vi "HFRR ADV v01.vi"() -> ()   [LabVIEW 2025] (continued)
        n280 = call "ELAPSED TIMER VI - Calibration.vi"("RESET"=w303, "PAUSE"=w303) -> ()  [unwired: 7 in, 3 out]
      }
      frame True {
        w306 = FALSE ("PAUSE")
        n281 = call "ELAPSED TIMER VI - Calibration.vi"("TARGET"=60.0, "RESET"=w306, "PAUSE"=w306) -> ("ELAPSED INDICATION"=w304:bool)  [unwired: 6 in, 2 out]
        n282 = case shown="False" w304 {
          frame False {
            n283 = local write "Friction Force Calibration Result Tab"(enum32{"Calibration Results", "Page 2"}."Calibration Results" ("Friction Force Calibration Result Tab")) -> ()
            n284 = property on="Friction Force Calibration Result Tab" class="TabCtl (strict)"("Visible"=FALSE) -> ()  [unwired: 2 in, 2 out]
          }
          frame True {
            n285 = stacked-sequence {
              frame #0 {
                n286 = local read "Friction"() -> (→"Friction cal":dbl)
                n287 = local write "run test Calibration"(FALSE ("run test Calibration")) -> ()
                n288 = local write "START TEMP"(FALSE ("START TEMP")) -> ()
              }
              frame #1 {
                n289 = Wait (ms)(milliseconds to wait=u32 1500) -> ()  [unwired: 1 out]
              }
              frame #2 {
                n290 = local write "Due Write"("VC;0") -> ()
              }
              frame #3 {
                n291 = Wait (ms)(milliseconds to wait=u32 1500) -> ()  [unwired: 1 out]
              }
              frame #4 {
                n292 = local write "Due Write"("VC;0") -> ()
              }
              frame #5 {
                n293 = property on="Friction Force Calibration Result Tab" class="TabCtl (strict)"("Visible"=TRUE) -> ()  [unwired: 2 in, 2 out]
                n294 = property on="Tab Control 6" class="TabCtl (strict)"("Visible"=FALSE) -> ()  [unwired: 2 in, 2 out]
              }
            }
          }
        }
      }
    }
    n295 = local read "Friction cal"() -> (w274:dbl)
    n296 = case shown="False" w278 {
      frame False {
        n297 = property on="Accept & Save" class="Bool (strict)"("DisabledEnum"=T20."Disabled" ("Disabled")) -> ()  [unwired: 2 in, 2 out]
        n298 = property on="Tab Control 5" class="TabCtl (strict)"("Value"=enum32{"OK", "NG"}."NG" ("Tab Control 5")) -> ()  [unwired: 2 in, 2 out]
      }
      frame True {
        n299 = property on="Accept & Save" class="Bool (strict)"("DisabledEnum"=T20."Enabled" ("Disabled")) -> ()  [unwired: 2 in, 2 out]
        n300 = property on="Tab Control 5" class="TabCtl (strict)"("Value"=enum32{"OK", "NG"}."OK" ("Tab Control 5")) -> ()  [unwired: 2 in, 2 out]
      }
    }
    n301 = Greater Or Equal?(x=w274, y="FF CAL EXCPTED VALUE") -> (x >= y?=w272:bool)
    n302 = case shown="False" w272 {
      selector: w272 -> [w285 w288]
      frame False {
        n303 = local write "FF PASS"(w285) -> ()
        n304 = local write "Friction Force result Tab"(enum32{"OK", "NG"}."NG" ("Friction Force result Tab")) -> ()
        n305 = property on="Accept & Save FF" class="Bool (strict)"("DisabledEnum"=T20."Disabled" ("Disabled")) -> ()  [unwired: 2 in, 2 out]
      }
      frame True {
        n306 = local write "Friction Force result Tab"(enum32{"OK", "NG"}."OK" ("Friction Force result Tab")) -> ()
        n307 = property on="Accept & Save FF" class="Bool (strict)"("DisabledEnum"=T20."Enabled" ("Disabled")) -> ()  [unwired: 2 in, 2 out]
        "FF PASS" <- w288
      }
    }
    n308 = local read "Quit"() -> (w284:bool)
  }
  n309 = while {
    stop <- w406 stop-if-true
    n310 = event shown="[13] \"Cal Password\": Value Change" {
      selector: _ -> [_ _ _ _ _ _ _ _ _ _ _ _ _ _ _ _ _ _ _ _ _ _ _ _ _ _ _ _ _ _ _ _ _ _ _ _ _ _ _ _ _ _ _ _ _ _ _ _ _ _ _ _ _ _ _ _ _]
      dyn-events: _ -> [_ _ _ _ _ _ _ _ _ _ _ _ _ _ _ _ _ _ _ _ _ _ _ _ _ _ _ _ _ _ _ _ _ _ _ _ _ _ _ _ _ _ _ _ _ _ _ _ _ _ _ _ _ _ _ _ _]
      timeout: 100 -> [_ _ _ _ _ _ _ _ _ _ _ _ _ _ _ _ _ _ _ _ _ _ _ _ _ _ _ _ _ _ _ _ _ _ _ _ _ _ _ _ _ _ _ _ _ _ _ _ _ _ _ _ _ _ _ _ _]
      tunnel: [FALSE FALSE FALSE _ FALSE _ _ _ _ _ _ _ _ _ _ _ _ _ _ _ _ _ _ _ _ _ _ _ _ _ _ _ _ _ _ _ _ _ _ _ _ _ _ _ _ _ _ _ _ _ _ _ _ _ _ _ TRUE] -> w406
      event Timeout {
        n311 = event-data() -> ()  [unwired: 1 in, 3 out]
        n312 = disable-structure shown="Disabled" {
          frame Disabled {
            n313 = local read "Auto Start Test"() -> (w420:bool)
            n314 = local read "RUN"() -> (w421:bool)
            n315 = Or(x=w421, y=w420) -> (x .or. y?=w419:bool)
            n316 = case shown="True" w419 {
              frame False {
                w422 = TRUE ("PAUSE")
                n317 = call "ELAPSED TIMER VI - abort test.vi"("RESET"=w422, "PAUSE"=w422) -> ()  [unwired: 7 in, 3 out]
              }
              frame True {
                n318 = local read "Stroke 2"() -> (w427:dbl)
                n319 = local read "FF 3"() -> (w429:dbl)
                n320 = Equal?(x=w427, y=0.95 ("Stroke 2")) -> (x = y?=w424:bool)
                n321 = Equal?(x=w429, y=0.0 ("FF 3")) -> (x = y?=w425:bool)
                n322 = Or(x=w425, y=w424) -> (x .or. y?=w423:bool)
                n323 = case shown="True" w423 {
                  selector: w423 -> [_ w434]
                  frame False {
                    w430 = TRUE ("PAUSE")
                    n324 = call "ELAPSED TIMER VI - abort test.vi"("RESET"=w430, "PAUSE"=w430) -> ()  [unwired: 7 in, 3 out]
                  }
                  frame True {
                    n325 = Not(x=w434) -> (.not. x?=w433:bool)
                    n326 = call "ELAPSED TIMER VI - abort test.vi"("TARGET"=60.0, "RESET"=w433, "PAUSE"=FALSE) -> ("ELAPSED INDICATION"=w431:bool)  [unwired: 6 in, 2 out]
                    n327 = case shown="True" w431 {
                      frame False {
                      }
                      frame True {
                        n328 = stacked-sequence {
                          frame #0 {
                            w436 = FALSE
                            n329 = local write "RUN"(w436) -> ()
                            n330 = local write "Auto Start Test"(w436) -> ()
                          }
                          frame #1 {
                            n331 = One Button Dialog(message="Test stopped due to a communication error. Reconnect the C1 and C2 cables.") -> ()  [unwired: 1 in, 1 out]
                          }
                        }
                      }
                    }
                  }
                }
              }
            }
          }
          frame Enabled {
          }
        }
        n332 = Get Date/Time In Seconds() -> (seconds since 1Jan1904=w417:timestamp)
        n333 = Format Into String(format string="%<%m/%d/%Y %I:%M:%S %p>T", w417) -> (resulting string=→"Time Stamp":string)  [unwired: 2 in, 1 out]
        n334 = local read "Service Password enable"() -> (w409:bool)
        n335 = local read "FILE"() -> (w414:string)
        n336 = call <vilib>:"Trim Whitespace.vi"("string"=w414) -> ("trimmed string"=w413:string)  [unwired: 1 in]
        n337 = String Length(string=w413) -> (length=w412:i32)
        n338 = Greater?(x=w412, y=1) -> (0:w410:bool)
        n339 = case shown="False" w410 {
          tunnel: w409 -> [w438 _]
          frame False {
            n340 = case shown="False" w438 {
              frame True {
                w439 = "Test Start In Service Mode" ("Tip Strip")
                w440 = T20."Enabled" ("Disabled")
                n341 = property on="Auto Start Test" class="Bool (strict)"("DisabledEnum"=w440, "TipStrip"=w439) -> ()  [unwired: 2 in, 2 out]
                n342 = property on="RUN" class="Bool (strict)"("DisabledEnum"=w440, "TipStrip"=w439) -> ()  [unwired: 2 in, 2 out]
              }
              frame False {
                w441 = "Enter File Name to Start Test" ("Tip Strip")
                w442 = T20."Disabled and Grayed Out" ("Disabled")
                n343 = property on="Auto Start Test" class="Bool (strict)"("DisabledEnum"=w442, "TipStrip"=w441) -> ()  [unwired: 2 in, 2 out]
                n344 = property on="RUN" class="Bool (strict)"("DisabledEnum"=w442, "TipStrip"=w441) -> ()  [unwired: 2 in, 2 out]
              }
            }
          }
          frame True {
            w443 = "" ("Tip Strip")
            w444 = T20."Enabled" ("Disabled")
            n345 = property on="Auto Start Test" class="Bool (strict)"("DisabledEnum"=w444, "TipStrip"=w443) -> ()  [unwired: 2 in, 2 out]
            n346 = property on="RUN" class="Bool (strict)"("DisabledEnum"=w444, "TipStrip"=w443) -> ()  [unwired: 2 in, 2 out]
          }
        }
      }
      event "RUN": Value Change {
        n347 = event-data() -> ()  [unwired: 1 in, 6 out]
        n348 = local read "RUN"() -> (w446:bool)
        n349 = case shown="False" w446 {
          frame False {
            n350 = flat-sequence {
              frame #0 {
                n351 = local write "START TEMP"(FALSE ("START TEMP")) -> ()
              }
              frame #1 {
                n352 = Wait (ms)(milliseconds to wait=u32 1500) -> ()  [unwired: 1 out]
              }
              frame #2 {
                n353 = local write "Humidity 2"(TRUE ("Humidity")) -> ()
              }
              frame #3 {
                n354 = local write "Due Write"("VC;0") -> ()
              }
              frame #4 {
                n355 = Wait (ms)(milliseconds to wait=u32 1500) -> ()  [unwired: 1 out]
              }
              frame #5 {
                w456 = T20."Enabled" ("Disabled")
                (unwired) T26."Imaging" ("Main Dashboard Buttons")
                (unwired) T22."Adv Scar" ("Main Tab")
                w458 = "" ("FILE")
                n356 = local write "measured_stroke"(0.0 ("measured_stroke")) -> ()
                n357 = local write "Due Write"("VC;0") -> ()
                n358 = local write "FILE"(w458) -> ()
                n359 = local write "Batch Ref Num :"(w458) -> ()
                n360 = local write "Fuel Discription :"(w458) -> ()
                n361 = local write "Main Tab"(T4."Adv Scar" ("Main Tab")) -> ()
                n362 = local write "Remarks :"(w458) -> ()
                n363 = local write "Main Dashboard Buttons"(T1."Imaging" ("Main Dashboard Buttons")) -> ()
                n364 = local write "TEST FILE NAM,E SAVED"(FALSE ("TEST FILE NAM,E SAVED")) -> ()
                n365 = property on="Stroke ( mm )" class="WFChart (strict)"("History Data"=cluster{"y":dbl, dbl, "y":dbl}[] []) -> ()  [unwired: 2 in, 2 out]
                n366 = property on="Auto Start Test" class="Bool (strict)"("Visible"=TRUE) -> ()  [unwired: 2 in, 2 out]
                n367 = property on="FRICVALZ 2" class="Bool (strict)"("DisabledEnum"=w456) -> ()  [unwired: 2 in, 2 out]
                n368 = property on="FRICVALZ 4" class="Bool (strict)"("DisabledEnum"=w456) -> ()  [unwired: 2 in, 2 out]
                n369 = property on="FRICVALZ 3" class="Bool (strict)"("DisabledEnum"=w456) -> ()  [unwired: 2 in, 2 out]
              }
            }
          }
          frame True {
            n370 = stacked-sequence {
              frame #0 {
                n371 = local write "FRICVALZ 4"(TRUE ("FRICVALZ 4")) -> ()
                n372 = local write "Due Write"("DAC;200") -> ()
              }
              frame #1 {
              }
              frame #2 {
              }
              frame #3 {
                n373 = Wait (ms)(milliseconds to wait=u32 1000) -> ()  [unwired: 1 out]
              }
              frame #4 {
                n374 = local write "Due Write"("VC;1") -> ()
              }
              frame #5 {
                n375 = Wait (ms)(milliseconds to wait=u32 1000) -> ()  [unwired: 1 out]
              }
              frame #6 {
                n376 = local write "Due Write"("VC;1") -> ()
              }
              frame #7 {
                n377 = Wait (ms)(milliseconds to wait=u32 1500) -> ()  [unwired: 1 out]
              }
              frame #8 {
                w469 = T20."Disabled" ("Disabled")
                n378 = property on="Auto Start Test" class="Bool (strict)"("Visible"=FALSE) -> ()  [unwired: 2 in, 2 out]
                n379 = local write "START TEMP"(TRUE ("START TEMP")) -> ()
                n380 = property on="FRICVALZ 2" class="Bool (strict)"("DisabledEnum"=w469) -> ()  [unwired: 2 in, 2 out]
                n381 = property on="FRICVALZ 4" class="Bool (strict)"("DisabledEnum"=w469) -> ()  [unwired: 2 in, 2 out]
                n382 = property on="FRICVALZ 3" class="Bool (strict)"("DisabledEnum"=w469) -> ()  [unwired: 2 in, 2 out]
              }
            }
          }
        }
      }
      event "run test Calibration": Value Change {
        n383 = event-data() -> ()  [unwired: 1 in, 6 out]
        n384 = local read "run test Calibration"() -> (w471:bool)
        n385 = case shown="False" w471 {
          frame False {
            n386 = flat-sequence {
              frame #0 {
                n387 = local write "START TEMP"(FALSE ("START TEMP")) -> ()
              }
              frame #1 {
                n388 = Wait (ms)(milliseconds to wait=u32 1500) -> ()  [unwired: 1 out]
              }
              frame #2 {
              }
              frame #3 {
                n389 = local write "Due Write"("VC;0") -> ()
              }
              frame #4 {
                n390 = Wait (ms)(milliseconds to wait=u32 1500) -> ()  [unwired: 1 out]
              }
              frame #5 {
                n391 = local write "Due Write"("VC;0") -> ()
                n392 = property on="Tab Control 6" class="TabCtl (strict)"("Visible"=FALSE) -> ()  [unwired: 2 in, 2 out]
                n393 = local write "Friction Force Calibration Result Tab"(enum32{"Calibration Results", "Page 2"}."Calibration Results" ("Friction Force Calibration Result Tab")) -> ()
                n394 = property on="Friction Force Calibration Result Tab" class="TabCtl (strict)"("Visible"=TRUE) -> ()  [unwired: 2 in, 2 out]
              }
            }
          }
          frame True {
            n395 = flat-sequence {
              frame #0 {
                n396 = local write "Due Write"("VC;1") -> ()
              }
              frame #1 {
                n397 = Wait (ms)(milliseconds to wait=u32 1000) -> ()  [unwired: 1 out]
              }
              frame #2 {
                n398 = local write "Due Write"("VC;1") -> ()
              }
              frame #3 {
                n399 = Wait (ms)(milliseconds to wait=u32 2000) -> ()  [unwired: 1 out]
              }
              frame #4 {
                n400 = local write "START TEMP"(TRUE ("START TEMP")) -> ()
                n401 = property on="Tab Control 6" class="TabCtl (strict)"("Visible"=TRUE) -> ()  [unwired: 2 in, 2 out]
                n402 = local write "Friction Force Calibration Result Tab"(enum32{"Calibration Results", "Page 2"}."Calibration Results" ("Friction Force Calibration Result Tab")) -> ()
              }
            }
          }
        }
      }
      event "Auto": Value Change {
        n403 = event-data() -> ()  [unwired: 1 in, 6 out]
        n404 = stacked-sequence {
          frame #0 {
            n405 = local write "FILE"("") -> ()
          }
          frame #1 {
            n406 = Get Date/Time In Seconds() -> (seconds since 1Jan1904=w492:timestamp)
            n407 = Format Into String(format string="%<%m_%d_%Y_%I_%M_%S_%p>T", w492) -> (resulting string=w491:string)  [unwired: 2 in, 1 out]
            n408 = local write "FILE"(w491) -> ()
          }
        }
        n409 = local read "Auto"() -> (w489:bool)
        n410 = Not(x=w489) -> (.not. x?=w488:bool)
        n411 = local write "Auto"(w488) -> ()
      }
      event "Auto Start Temp": Value Change {
        n412 = event-data() -> ()  [unwired: 1 in, 6 out]
        n413 = local read "Auto Start Test"() -> (w495:bool)
        n414 = case shown="False" w495 {
          frame False {
            n415 = stacked-sequence {
              frame #0 {
                n416 = local write "START TEMP"(FALSE ("START TEMP")) -> ()
              }
              frame #1 {
                n417 = Wait (ms)(milliseconds to wait=u32 2000) -> ()  [unwired: 1 out]
              }
              frame #2 {
                n418 = local write "Due Write"("VC;0") -> ()
              }
              frame #3 {
                n419 = Wait (ms)(milliseconds to wait=u32 2000) -> ()  [unwired: 1 out]
              }
              frame #4 {
                w506 = T20."Enabled" ("Disabled")
                (unwired) T26."Imaging" ("Main Dashboard Buttons")
                w507 = "" ("FILE")
                n420 = local write "Main Tab"(T4."Adv Scar" ("Main Tab")) -> ()
                n421 = local write "measured_stroke"(0.0 ("measured_stroke")) -> ()
                n422 = local write "Main Dashboard Buttons"(T1."Imaging" ("Main Dashboard Buttons")) -> ()
                n423 = property on="RUN" class="Bool (strict)"("Visible"=TRUE) -> ()  [unwired: 2 in, 2 out]
                n424 = local write "Due Write"("VC;0") -> ()
                n425 = local write "Humidity 2"(TRUE ("Humidity")) -> ()
                n426 = local write "TEST FILE NAM,E SAVED"(FALSE ("TEST FILE NAM,E SAVED")) -> ()
                n427 = local write "Fuel Discription :"(w507) -> ()
                n428 = local write "Batch Ref Num :"(w507) -> ()
                n429 = local write "Remarks :"(w507) -> ()
                n430 = local write "FILE"(w507) -> ()
                n431 = property on="FRICVALZ 2" class="Bool (strict)"("DisabledEnum"=w506) -> ()  [unwired: 2 in, 2 out]
                n432 = property on="FRICVALZ 4" class="Bool (strict)"("DisabledEnum"=w506) -> ()  [unwired: 2 in, 2 out]
                n433 = property on="FRICVALZ 3" class="Bool (strict)"("DisabledEnum"=w506) -> ()  [unwired: 2 in, 2 out]
              }
            }
          }
          frame True {
            n434 = stacked-sequence {
              frame #0 {
                n435 = local write "Due Write"("DAC;200") -> ()
              }
              frame #1 {
                n436 = Wait (ms)(milliseconds to wait=u32 1000) -> ()  [unwired: 1 out]
              }
              frame #2 {
              }
              frame #3 {
              }
              frame #4 {
                n437 = local write "Due Write"("VC;1") -> ()
              }
              frame #5 {
                n438 = Wait (ms)(milliseconds to wait=u32 1000) -> ()  [unwired: 1 out]
              }
              frame #6 {
                n439 = local write "Due Write"("VC;1") -> ()
              }
              frame #7 {
                n440 = Wait (ms)(milliseconds to wait=u32 1500) -> ()  [unwired: 1 out]
              }
              frame #8 {
                w516 = T20."Disabled" ("Disabled")
                n441 = property on="RUN" class="Bool (strict)"("Visible"=FALSE) -> ()  [unwired: 2 in, 2 out]
                n442 = property on="FRICVALZ 2" class="Bool (strict)"("DisabledEnum"=w516) -> ()  [unwired: 2 in, 2 out]
                n443 = property on="FRICVALZ 4" class="Bool (strict)"("DisabledEnum"=w516) -> ()  [unwired: 2 in, 2 out]
                n444 = property on="FRICVALZ 3" class="Bool (strict)"("DisabledEnum"=w516) -> ()  [unwired: 2 in, 2 out]
                "START TEMP" <- TRUE
              }
            }
          }
        }
      }
      event "FILE", "USERNAME", "USER ID": Mouse Enter {
        n445 = event-data() -> ()  [unwired: 1 in, 4 out]
        n446 = dll-call lib="kernel32.dll" fn="Wow64DisableWow64FsRedirection"("OldValue"=0) -> (error out=w523:errorcluster, "OldValue"=w521:i32)  [unwired: 4 in, 1 out]
        n447 = call <vilib>:"System Exec.vi"("run minimized? (F)"=TRUE, "error in (no error)"=w523, "command line"="C:\\Program Files\\Common Files\\Microsoft Shared\\Ink\\TabTip.exe") -> ("error out"=w522:errorcluster)  [unwired: 5 in, 3 out]
        n448 = dll-call lib="kernel32.dll" fn="Wow64EnableWow64FsRedirection"(error in=w522, "OldValue"=w521) -> ()  [unwired: 4 in, 2 out]
      }
      event "EDIT": Value Change {
        n449 = event-data() -> ()  [unwired: 1 in, 6 out]
        n450 = local read "EDIT"() -> (w524:bool)
        n451 = case shown="False" w524 {
          frame False {
            n452 = control-ref of="This VI"() -> (w541:refnum<vi>)
            n453 = property class="VI"(reference=w541) -> (reference out=w532:refnum<vi>, error out=w536:errorcluster, "Panel"=w540:refnum<vi>)  [unwired: 1 in]
            n454 = property class="Pnl"(reference=w540, error in=w536) -> (reference out=w534:refnum<vi>, error out=w537:errorcluster, "Panes[]"=w539:refnum<vi>[])
            n455 = for {
              tunnel: w539 -> [w547] mode=indexing
              tunnel: T25."Always Off" ("Horizontal Scrollbar Visibility") -> [w546]
              tunnel: w537 -> [w543]
              tunnel: [w542] -> w535
              n456 = property class="Pane"(reference=w547, error in=w543, "HorizScrollbarVisibility"=w546) -> (reference out=w544:refnum<vi>, error out=w545:errorcluster)
              n457 = Close Reference(reference=w544, error in (no error)=w545) -> (error out=w542:errorcluster)
            }
            n458 = Close Reference(reference=w534, error in (no error)=w535) -> (error out=w533:errorcluster)
            n459 = Close Reference(reference=w532, error in (no error)=w533) -> (error out=w527:errorcluster)
            "error out 7" <- w527
            n460 = call <vilib>:"Clear Errors.vi"("error in (no error)"=w527) -> ("error out"=w526:errorcluster)  [unwired: 5 in, 1 out]
            n461 = local write "Service Password enable"(FALSE ("Service Password enable")) -> ()
            n462 = call <userlib>:"Fit VI window to Largest Dec.vi"("error in (no error)"=w526, "border spacing (2 px)"=1) -> ("error out"=w531:errorcluster, "dup VI Ref"=w529:refnum<vi>)  [unwired: 4 in]
            n463 = invoke on="Invoke Node" class="VI" method="FP.Run-Time Position.Maximized"(reference=w529, error in=w531) -> (error out=w530:errorcluster)  [unwired: 2 in, 3 out]
            n464 = call <vilib>:"Clear Errors.vi"("error in (no error)"=w530) -> ()  [unwired: 5 in, 2 out]
          }
          frame True {
          }
        }
      }
      event "Heater Button": Value Change {
        n465 = event-data() -> ()  [unwired: 1 in, 6 out]
        n466 = local read "Heater Button"() -> (w548:bool)
        n467 = case shown="True" w548 {
          frame True {
            n468 = stacked-sequence {
              frame #0 {
                n469 = Wait (ms)(milliseconds to wait=u32 1500) -> ()  [unwired: 1 out]
              }
              frame #1 {
                n470 = local read "Set Temp"() -> (w550:dbl)
                n471 = Number To Fractional String(number=w550, precision (6)=i16 2) -> (F-format string=w553:string)  [unwired: 2 in]
                n472 = Concatenate Strings("ST;" ("Command"), w553) -> (w552:string)
                n473 = local write "Due Write"(w552) -> ()
              }
              frame #2 {
                n474 = Wait (ms)(milliseconds to wait=u32 1500) -> ()  [unwired: 1 out]
              }
              frame #3 {
                n475 = local write "Due Write"("HE;1" ("Command")) -> ()
              }
              frame #4 {
                n476 = Wait (ms)(milliseconds to wait=u32 1500) -> ()  [unwired: 1 out]
              }
              frame #5 {
                n477 = stacked-sequence {
                  frame #0 {
                    n478 = Wait (ms)(milliseconds to wait=u32 1500) -> ()  [unwired: 1 out]
                  }
                  frame #1 {
                    n479 = local read "Set Temp"() -> (w559:dbl)
                    n480 = Number To Fractional String(number=w559, precision (6)=i16 2) -> (F-format string=w562:string)  [unwired: 2 in]
                    n481 = Concatenate Strings("ST;" ("Command"), w562) -> (w561:string)
                    n482 = local write "Due Write"(w561) -> ()
                  }
                  frame #2 {
                    n483 = Wait (ms)(milliseconds to wait=u32 1500) -> ()  [unwired: 1 out]
                  }
                  frame #3 {
                    n484 = local write "Due Write"("HE;1" ("Command")) -> ()
                  }
                  frame #4 {
                    n485 = Wait (ms)(milliseconds to wait=u32 1500) -> ()  [unwired: 1 out]
                  }
                }
              }
            }
          }
          frame False {
            n486 = stacked-sequence {
              frame #0 {
                n487 = Wait (ms)(milliseconds to wait=u32 1500) -> ()  [unwired: 1 out]
              }
              frame #1 {
                n488 = Concatenate Strings("ST;" ("Command"), "0" ("string")) -> (w569:string)
                n489 = local write "Due Write"(w569) -> ()
              }
              frame #2 {
                n490 = Wait (ms)(milliseconds to wait=u32 1500) -> ()  [unwired: 1 out]
              }
              frame #3 {
                n491 = local write "Due Write"("HE;0" ("Command")) -> ()
              }
              frame #4 {
                n492 = Wait (ms)(milliseconds to wait=u32 1500) -> ()  [unwired: 1 out]
              }
            }
          }
        }
      }
      event "Headen Service Button": Value Change {
        n493 = event-data() -> ()  [unwired: 1 in, 6 out]
        n494 = local read "Headen Service Button"() -> (w574:bool)
        n495 = case shown="True" w574 {
          frame False {
            n496 = property on="Password 3" class="Clust (strict)"("Visible"=FALSE) -> ()  [unwired: 2 in, 2 out]
            n497 = property on="Service Password Log" class="Str"("Visible"=FALSE) -> ()  [unwired: 2 in, 2 out]
          }
          frame True {
            n498 = flat-sequence {
              tunnel: [w580] -> w577
              tunnel: w577 -> [w581]
              frame #0 {
                n499 = property on="Password 3" class="Clust (strict)"("Visible"=TRUE) -> ()  [unwired: 2 in, 2 out]
                n500 = property on="Service Password Log" class="Str"("Visible"=TRUE) -> ()  [unwired: 2 in, 2 out]
              }
              frame #1 {
                n501 = call "DIALOG BOX HFRR ADV.vi"() -> ("Continue"=w580:bool)  [unwired: 8 in, 2 out]
              }
              frame #2 {
                n502 = case shown="True" w581 {
                  frame True {
                    n503 = property on="Password 3" class="Clust (strict)"("Visible"=TRUE) -> ()  [unwired: 2 in, 2 out]
                    n504 = property on="Service Password Log" class="Str"("Visible"=TRUE) -> ()  [unwired: 2 in, 2 out]
                  }
                  frame False {
                    n505 = property on="Password 3" class="Clust (strict)"("Visible"=FALSE) -> ()  [unwired: 2 in, 2 out]
                    n506 = property on="Service Password Log" class="Str"("Visible"=FALSE) -> ()  [unwired: 2 in, 2 out]
                  }
                }
              }
            }
          }
        }
      }
      event "Password 3.Service Password": Value Change {
        n507 = event-data() -> ()  [unwired: 1 in, 6 out]
        n508 = Unbundle By Name("Password 3") -> ("Service Password"=w588:string)
        n509 = call <vilib>:"Trim Whitespace.vi"("string"=w588) -> ("trimmed string"=w586:string)  [unwired: 1 in]
        n510 = Equal?(x=w586, y="Service@123") -> (x = y?=w587:bool)
        n511 = case shown="True" w587 {
          selector: w587 -> [w592 w595]
          frame False {
            w591 = FALSE
            n512 = local write "Service Password enable"(w592) -> ()
            n513 = property on="Service Password Log" class="Str"("Visible"=TRUE) -> ()  [unwired: 2 in, 2 out]
            n514 = property on="Service Left" class="Bool (strict)"("Visible"=w591) -> ()  [unwired: 2 in, 2 out]
            n515 = property on="Service Right" class="Bool (strict)"("Visible"=w591) -> ()  [unwired: 2 in, 2 out]
            n516 = property on="Service Bottom" class="Bool (strict)"("Visible"=w591) -> ()  [unwired: 2 in, 2 out]
          }
          frame True {
            w594 = TRUE
            n517 = property on="Service Password Log" class="Str"("Visible"=FALSE) -> ()  [unwired: 2 in, 2 out]
            n518 = property on="Service Left" class="Bool (strict)"("Visible"=w594) -> ()  [unwired: 2 in, 2 out]
            n519 = property on="Service Right" class="Bool (strict)"("Visible"=w594) -> ()  [unwired: 2 in, 2 out]
            n520 = property on="Service Bottom" class="Bool (strict)"("Visible"=w594) -> ()  [unwired: 2 in, 2 out]
            "Service Password enable" <- w595
          }
        }
      }
      event "Sign In": Value Change {
        w597 = FALSE ("Visible")
        n521 = event-data() -> ()  [unwired: 1 in, 6 out]
        n522 = property on="About" class="Clust (strict)"("Visible"=w597) -> ()  [unwired: 2 in, 2 out]
        n523 = property on="Password 3" class="Clust (strict)"("Visible"=w597) -> ()  [unwired: 2 in, 2 out]
        n524 = property on="Service Password Log" class="Str"("Visible"=FALSE) -> ()  [unwired: 2 in, 2 out]
      }
      event "Info": Value Change {
        n525 = event-data() -> ()  [unwired: 1 in, 6 out]
        n526 = local read "Operating System"() -> (w602:string)
        n527 = local read "Firmware Version"() -> (w603:string)
        n528 = local read "Instrument Serial"() -> (w601:string)
        n529 = local read "Workorder"() -> (w605:string)
        n530 = local write "Info"(FALSE) -> ()
        n531 = local read "Runtime"() -> (w604:string)
        n532 = local read "Version"() -> (w606:string)
        n533 = local read "version"() -> (w607:string)
        n534 = Insert Into Array(array=string[] [], new element #1=w607, new element #2=w606, new element #3=w605, new element #4=w604, new element #5=w603, new element #6=w602, new element #7=w601) -> (w600:string[])  [unwired: 1 in]
        n535 = call "ABOUT SCREEN ADV NEW.vi"("Array"=w600) -> ()  [unwired: 10 in, 1 out]
      }
      event "Calibration": Value Change {
        n536 = event-data() -> ()  [unwired: 1 in, 6 out]
        n537 = local read "Calibration"() -> (w610:bool)
        n538 = case shown="False" w610 {
          frame False {
            n539 = property on="Calibration 2" class="TabCtl (strict)"("Visible"=FALSE) -> ()  [unwired: 2 in, 2 out]
            n540 = local write "Cal Password"("" ("Cal Password")) -> ()
          }
          frame True {
            n541 = property on="Calibration 2" class="TabCtl (strict)"("Visible"=TRUE) -> ()  [unwired: 2 in, 2 out]
            n542 = local write "Cal Password"("" ("Cal Password")) -> ()
          }
        }
        n543 = property on="Wrong Password" class="Str"("Visible"=FALSE) -> ()  [unwired: 2 in, 2 out]
      }
      event "Cal Password": Value Change {
        n544 = event-data() -> ()  [unwired: 1 in, 6 out]
        n545 = local read "Cal Password"() -> (w618:string)
        n546 = call <vilib>:"Trim Whitespace.vi"("string"=w618) -> ("trimmed string"=w617:string)  [unwired: 1 in]
        n547 = Equal?(x=w617, y="Cal@321") -> (x = y?=w615:bool)
        n548 = case shown="True" w615 {
          frame False {
            n549 = property on="Wrong Password" class="Str"("Visible"=TRUE) -> ()  [unwired: 2 in, 2 out]
          }
          frame True {
            n550 = property on="Wrong Password" class="Str"("Visible"=FALSE) -> ()  [unwired: 2 in, 2 out]
            n551 = local write "Main Tab"(T4."About" ("Main Tab")) -> ()
            n552 = local write "Cal Password"("" ("Cal Password")) -> ()
            n553 = local write "Main Dashboard Buttons"(T1."About" ("Main Dashboard Buttons")) -> ()
            n554 = property on="Calibration 2" class="TabCtl (strict)"("Visible"=FALSE) -> ()  [unwired: 2 in, 2 out]
            n555 = local write "Calibration"(FALSE ("Calibration")) -> ()
          }
        }
      }
      event "Calibration Selection": Value Change {
        n556 = event-data() -> ()  [unwired: 1 in, 6 out]
        n557 = local read "Calibration Selection"() -> (w627:T10)
        n558 = case shown="\"Stroke Calibration\"" w627 {
          tunnel: [T9."Stroke" ("Main Calibration Tab") T9."Friction" ("Main Calibration Tab") T9."Main" ("Main Calibration Tab") T9."Temperature" ("Main Calibration Tab")] -> w626
          frame "Stroke Calibration" {
          }
          frame "Friction Force Calibration" {
          }
          frame Default {
          }
          frame "Temperature Calibration" {
          }
        }
        n559 = local write "Main Calibration Tab"(w626) -> ()
      }
      event "Back Stroke": Value Change {
        n560 = event-data() -> ()  [unwired: 1 in, 6 out]
        n561 = local write "Main Stroke Tab"(T11."Step 1" ("Main Stroke Tab")) -> ()
        n562 = local write "Main Calibration Tab"(T9."Main" ("Main Calibration Tab")) -> ()
        n563 = local write "Back Stroke"(FALSE ("Back Stroke")) -> ()
        n564 = local write "Calibration Selection"(T10."Default" ("Calibration Selection")) -> ()
      }
      event "Step 2 Back": Value Change {
        n565 = event-data() -> ()  [unwired: 1 in, 6 out]
        n566 = local write "Main Stroke Tab"(T11."Step 1" ("Main Stroke Tab")) -> ()
        n567 = local write "Step 2 Back"(FALSE ("Back Stroke")) -> ()
        n568 = local write "Calibration Selection"(T10."Default" ("Calibration Selection")) -> ()
      }
      event "Step 3 Back": Value Change {
        n569 = event-data() -> ()  [unwired: 1 in, 6 out]
        n570 = local write "Main Stroke Tab"(T11."Step 2" ("Main Stroke Tab")) -> ()
        n571 = local write "Step 3 Back"(FALSE ("Back Stroke")) -> ()
        n572 = local write "Calibration Selection"(T10."Default" ("Calibration Selection")) -> ()
      }
      event "Step 4 Back": Value Change {
        n573 = event-data() -> ()  [unwired: 1 in, 6 out]
        n574 = local write "Main Stroke Tab"(T11."Step 3" ("Main Stroke Tab")) -> ()
        n575 = local write "Step 4 Back"(FALSE ("Back Stroke")) -> ()
        n576 = local write "Calibration Selection"(T10."Default" ("Calibration Selection")) -> ()
      }
      event "Step 5 Back": Value Change {
        n577 = event-data() -> ()  [unwired: 1 in, 6 out]
        n578 = local write "Main Stroke Tab"(T11."Step 4" ("Main Stroke Tab")) -> ()
        n579 = local write "Step 5 Back"(FALSE ("Back Stroke")) -> ()
        n580 = local write "Calibration Selection"(T10."Default" ("Calibration Selection")) -> ()
      }
      event "Step 6 Back": Value Change {
        n581 = event-data() -> ()  [unwired: 1 in, 6 out]
        n582 = local write "Main Stroke Tab"(T11."Step 5" ("Main Stroke Tab")) -> ()
        n583 = local write "Step 6 Back"(FALSE ("Back Stroke")) -> ()
        n584 = local write "Calibration Selection"(T10."Default" ("Calibration Selection")) -> ()
      }
      event "Back Stroke step 7": Value Change {
        n585 = event-data() -> ()  [unwired: 1 in, 6 out]
        n586 = local write "Main Stroke Tab"(T11."Step 5" ("Main Stroke Tab")) -> ()
        n587 = local write "Back Stroke step 7"(FALSE ("Back Stroke")) -> ()
        n588 = local write "Calibration Selection"(T10."Default" ("Calibration Selection")) -> ()
      }
      event "Back Stroke step 8": Value Change {
        n589 = event-data() -> ()  [unwired: 1 in, 6 out]
        n590 = local write "Main Stroke Tab"(T11."Step 7" ("Main Stroke Tab")) -> ()
        n591 = local write "Back Stroke step 8"(FALSE ("Back Stroke")) -> ()
        n592 = local write "Calibration Selection"(T10."Default" ("Calibration Selection")) -> ()
      }
      event "Back Stroke 8": Value Change {
        n593 = event-data() -> ()  [unwired: 1 in, 6 out]
        n594 = local write "MOVE CARRIAGE TO"(1.0 ("MOVE CARRIAGE TO")) -> ()
        n595 = local write "Main Stroke Tab"(T11."Step 1" ("Main Stroke Tab")) -> ()
        n596 = local write "Calibration Selection"(T10."Default" ("Calibration Selection")) -> ()
        n597 = local write "Back Stroke 8"(FALSE ("Back Stroke 8")) -> ()
      }
      event "Continue Stroke": Value Change {
        n598 = event-data() -> ()  [unwired: 1 in, 6 out]
        n599 = local write "Main Stroke Tab"(T11."Step 2" ("Main Stroke Tab")) -> ()
        n600 = local write "Continue Stroke"(FALSE ("Continue Stroke")) -> ()
      }
      event "Continue Stroke step 2": Value Change {
        n601 = event-data() -> ()  [unwired: 1 in, 6 out]
        n602 = local write "Main Stroke Tab"(T11."Step 3" ("Main Stroke Tab")) -> ()
        n603 = local write "Continue Stroke step 2"(FALSE ("Continue Stroke")) -> ()
      }
      event "Continue Stroke step 3": Value Change {
        n604 = event-data() -> ()  [unwired: 1 in, 6 out]
        n605 = local write "Main Stroke Tab"(T11."Step 4" ("Main Stroke Tab")) -> ()
        n606 = local write "Continue Stroke step 3"(FALSE ("Continue Stroke")) -> ()
      }
      event "Continue Stroke step 4": Value Change {
        n607 = event-data() -> ()  [unwired: 1 in, 6 out]
        n608 = local write "Main Stroke Tab"(T11."Step 5" ("Main Stroke Tab")) -> ()
        n609 = local write "Continue Stroke step 4"(FALSE ("Continue Stroke")) -> ()
      }
      event "Continue Stroke step 5": Value Change {
        n610 = event-data() -> ()  [unwired: 1 in, 6 out]
        n611 = local write "Main Stroke Tab"(T11."Step 7" ("Main Stroke Tab")) -> ()
        n612 = local write "Continue Stroke step 5"(FALSE ("Continue Stroke")) -> ()
      }
      event "Continue Stroke step 6": Value Change {
        n613 = event-data() -> ()  [unwired: 1 in, 6 out]
        n614 = local write "Main Stroke Tab"(T11."Step 7" ("Main Stroke Tab")) -> ()
        n615 = local write "Continue Stroke step 6"(FALSE ("Continue Stroke")) -> ()
      }
      event "Continue Stroke step 7": Value Change {
        w675 = FALSE ("0.2mm")
        n616 = event-data() -> ()  [unwired: 1 in, 6 out]
        n617 = local write "0.4 mm"(w675) -> ()
        n618 = local write "0.6 mm"(w675) -> ()
        n619 = local write "1.0 mm"(w675) -> ()
        n620 = local write "1.2 mm"(w675) -> ()
        n621 = local write "0.2 2"(w675) -> ()
        n622 = local write "0.4 2"(w675) -> ()
        n623 = local write "0.6 2"(w675) -> ()
        n624 = local write "0.8 2"(w675) -> ()
        n625 = local write "1.0 2"(w675) -> ()
        n626 = local write "1.2"(w675) -> ()
        n627 = local write "0.2mm"(w675) -> ()
        n628 = local write "0.8mm"(w675) -> ()
        n629 = local write "Main Stroke Tab"(T11."Step 8" ("Main Stroke Tab")) -> ()
        n630 = local write "Continue Stroke step 7"(FALSE ("Continue Stroke")) -> ()
        n631 = local write "Stroke Test Complete"(T12."Test Progress" ("Stroke Test Complete")) -> ()
        "Position Measurment Temp" <- 4.0 ("Position Measurment Temp")
        "Calibration Tare" <- TRUE ("Calibration Tare")
        "MOVE CARRIAGE TO" <- 1.0 ("MOVE CARRIAGE TO")
      }
      event "Continue Stroke step 8": Value Change {
        n632 = event-data() -> ()  [unwired: 1 in, 6 out]
        n633 = local read "LVDT STROKE  Calibration"() -> (w680:dbl)
        n634 = local read "Position Measurment Temp"() -> (w681:dbl)
        n635 = case shown="7" w681 {
          selector: w681 -> [w686 w691 w696 w701 _ w709 w712 w713]
          tunnel: w680 -> [w682 w687 w692 w697 w703 w706 _ _]
          frame 0, Default {
            w684 = TRUE ("0.2mm")
            n636 = Increment(x=w686) -> (x+1=w685:i32)
            n637 = local write "Position Measurment Temp"(w685) -> ()
            n638 = local write "0.2mm"(w684) -> ()
            n639 = local write "0.2 2"(w684) -> ()
            n640 = local write "MOVE CARRIAGE TO"(1.0 ("MOVE CARRIAGE TO")) -> ()
            "Calibration 0.2" <- w682
          }
          frame 1 {
            w689 = TRUE ("0.4 mm")
            n641 = Increment(x=w691) -> (x+1=w690:i32)
            n642 = local write "Calibration 0.4"(w687) -> ()
            n643 = local write "Position Measurment Temp"(w690) -> ()
            n644 = local write "0.4 mm"(w689) -> ()
            n645 = local write "MOVE CARRIAGE TO"(0.6 ("MOVE CARRIAGE TO")) -> ()
            n646 = local write "0.4 2"(w689) -> ()
          }
          frame 2 {
            w694 = TRUE ("0.6 mm")
            n647 = Increment(x=w696) -> (x+1=w695:i32)
            n648 = local write "Calibration 0.6"(w692) -> ()
            n649 = local write "Position Measurment Temp"(w695) -> ()
            n650 = local write "0.6 2"(w694) -> ()
            n651 = local write "0.6 mm"(w694) -> ()
            n652 = local write "MOVE CARRIAGE TO"(0.8 ("MOVE CARRIAGE TO")) -> ()
          }
          frame 3 {
            w698 = TRUE ("0.6 mm")
            n653 = Increment(x=w701) -> (x+1=w700:i32)
            n654 = local write "Position Measurment Temp"(w700) -> ()
            n655 = local write "MOVE CARRIAGE TO"(1.0 ("MOVE CARRIAGE TO")) -> ()
            n656 = local write "0.8mm"(w698) -> ()
            n657 = local write "0.8 2"(w698) -> ()
            "Calibration 0.8" <- w697
          }
          frame 4 {
            w704 = TRUE ("0.6 mm")
            n658 = local write "Position Measurment Temp"(6.0 ("Position Measurment Temp")) -> ()
            n659 = local write "MOVE CARRIAGE TO"(1.0 ("MOVE CARRIAGE TO")) -> ()
            n660 = local write "1.0 mm"(w704) -> ()
            n661 = local write "1.0 2"(w704) -> ()
            "Calibration 1.0" <- w703
          }
          frame 5 {
            w707 = TRUE ("0.6 mm")
            n662 = Increment(x=w709) -> (x+1=w708:i32)
            n663 = local write "Position Measurment Temp"(w708) -> ()
            n664 = local write "1.2 mm"(w707) -> ()
            n665 = local write "1.2"(w707) -> ()
            "Calibration 1.2" <- w706
          }
          frame 6 {
            n666 = Increment(x=w712) -> (x+1=w711:i32)
            n667 = local write "Position Measurment Temp"(w711) -> ()
            n668 = local write "Stroke Test Complete"(T12."Stroke Points Completed" ("Stroke Test Complete")) -> ()
          }
          frame 7 {
            n669 = stacked-sequence {
              tunnel: w713 -> [w714 _ _]
              frame #0 {
                n670 = Increment(x=w714) -> (x+1=w715:i32)
                n671 = local write "Main Stroke Tab"(T11."Step 9" ("Main Stroke Tab")) -> ()
                n672 = local write "Position Measurment Temp"(w715) -> ()
                n673 = Insert Into Array(array=dbl[] [], new element #1=0.2 ("new element/subarray"), new element #2=0.4 ("new element/subarray"), new element #3=0.6 ("new element/subarray"), new element #4=0.8 ("new element/subarray"), new element #5=1.0 ("new element/subarray"), new element #6=1.2 ("new element/subarray")) -> (→"1D stroke":dbl[])  [unwired: 1 in]
                n674 = local read "Calibration 0.2"() -> (w722:dbl)
                n675 = local read "Calibration 0.4"() -> (w721:dbl)
                n676 = local read "Calibration 0.6"() -> (w720:dbl)
                n677 = local read "Calibration 0.8"() -> (w719:dbl)
                n678 = local read "Calibration 1.0"() -> (w718:dbl)
                n679 = local read "Calibration 1.2"() -> (w717:dbl)
                n680 = Insert Into Array(array=dbl[] [], new element #1=w722, new element #2=w721, new element #3=w720, new element #4=w719, new element #5=w718, new element #6=w717) -> (→"Calibrated Voltage Value":dbl[])  [unwired: 1 in]
              }
              frame #1 {
                n681 = local read "calibration values"() -> (w745:dbl[])
                n682 = local read "Calibrated Voltage Value"() -> (w747:dbl[])
                n683 = Index Array(array=w745, index #1=1 ("index"), index #2=3 ("index"), index #3=5 ("index"), index #4=7 ("index"), index #5=9 ("index"), index #6=11 ("index")) -> (element #1=w738:dbl, element #2=w737:dbl, element #3=w736:dbl, element #4=w735:dbl, element #5=w734:dbl, element #6=w733:dbl)
                n684 = local read "1D stroke"() -> (w748:dbl[])
                n685 = for {
                  tunnel: [w757] -> w746 mode=indexing
                  tunnel: w748 -> [w756] mode=indexing
                  tunnel: w747 -> [w755] mode=indexing
                  tunnel: w738 -> [w754]
                  tunnel: w737 -> [w753]
                  tunnel: w736 -> [w752]
                  tunnel: w735 -> [w751]
                  tunnel: w734 -> [w750]
                  tunnel: w733 -> [w749]
                  n686 = formula code="if (stroke == 0.2)\n{\n    if ((voltage >= REF_02 - 0.2) && (voltage <= REF_02 + 0.2))\n        status = 1;\n    else\n        status = 0;\n}\nelse if (stroke == 0.4)\n{\n    if ((voltage >= REF_04 - 0.2) && (voltage <= REF_04 + 0.2))\n        status = 1;\n    else\n        status = 0;\n}\nelse if (stroke == 0.6)\n{\n    if ((voltage >= REF_06 - 0.2) && (voltage <= REF_06 + 0.2))\n        status = 1;\n    else\n        status = 0;\n}\nelse if (stroke == 0.8)\n{\n    if ((voltage >= REF_08 - 0.2) && (voltage <= REF_08 + 0.2))\n        status = 1;\n    else\n        status = 0;\n}\nelse if (stroke == 1.0)\n{\n    if ((voltage >= REF_10 - 1) && (voltage <= REF_10 + 1))\n        status = 1;\n    else\n        status = 0;\n}\nelse if (stroke == 1.2)\n{\n    if ((voltage >= REF_12 - 0.2) && (voltage <= REF_12 + 0.2))\n        status = 1;\n    else\n        status = 0;\n}\nelse\n{\n    status = 0;\n}"("stroke"=w756, "voltage"=w755, "REF_02"=w754, "REF_04"=w753, "REF_06"=w752, "REF_08"=w751, "REF_10"=w750, "REF_12"=w749) -> ("status"=w757:dbl)
                }
                "Status" <- w746
              }
              frame #2 {
                w764 = 1.0
                n687 = local read "Status"() -> (w771:dbl[])
                n688 = Index Array(array=w771) -> (element #1=w770:dbl, element #2=w769:dbl, element #3=w768:dbl, element #4=w767:dbl, element #5=w766:dbl, element #6=w765:dbl)  [unwired: 6 in]
                n689 = Equal?(x=w769, y=w764) -> (x = y?=w762:bool)
                n690 = Equal?(x=w768, y=w764) -> (x = y?=w761:bool)
                n691 = Equal?(x=w767, y=w764) -> (x = y?=w760:bool)
                n692 = Equal?(x=w766, y=w764) -> (x = y?=w759:bool)
                n693 = Equal?(x=w765, y=w764) -> (x = y?=w758:bool)
                n694 = Equal?(x=w770, y=w764) -> (x = y?=w763:bool)
                n695 = case shown="True" w763 {
                  selector: w763 -> [w782 w783]
                  frame True {
                    n696 = local write "Point 1 - 0.2 mm"(w782) -> ()
                    n697 = property on="Point 1 - 0.2 mm" class="Bool"("Caption.Visible"=w782) -> ()  [unwired: 2 in, 2 out]
                  }
                  frame False {
                    n698 = local write "Point 1 - 0.2 mm"(w783) -> ()
                    n699 = property on="Point 1 - 0.2 mm" class="Bool"("Caption.Visible"=w783) -> ()  [unwired: 2 in, 2 out]
                  }
                }
                n700 = case shown="True" w762 {
                  selector: w762 -> [w780 w781]
                  frame True {
                    n701 = local write "Point 2 - 0.4 mm"(w780) -> ()
                    n702 = property on="Point 2 - 0.4 mm" class="Bool"("Caption.Visible"=w780) -> ()  [unwired: 2 in, 2 out]
                  }
                  frame False {
                    n703 = local write "Point 2 - 0.4 mm"(w781) -> ()
                    n704 = property on="Point 2 - 0.4 mm" class="Bool"("Caption.Visible"=w781) -> ()  [unwired: 2 in, 2 out]
                  }
                }
                n705 = case shown="True" w759 {
                  selector: w759 -> [w774 w775]
                  frame True {
                    n706 = local write "Point 5 - 1.0 mm"(w774) -> ()
                    n707 = property on="Point 5 - 1.0 mm" class="Bool"("Caption.Visible"=w774) -> ()  [unwired: 2 in, 2 out]
                  }
                  frame False {
                    n708 = local write "Point 5 - 1.0 mm"(w775) -> ()
                    n709 = property on="Point 5 - 1.0 mm" class="Bool"("Caption.Visible"=w775) -> ()  [unwired: 2 in, 2 out]
                  }
                }
                n710 = case shown="True" w761 {
                  selector: w761 -> [w778 w779]
                  frame True {
                    n711 = local write "Point 3 - 0.6 mm"(w778) -> ()
                    n712 = property on="Point 3 - 0.6 mm" class="Bool"("Caption.Visible"=w778) -> ()  [unwired: 2 in, 2 out]
                  }
                  frame False {
                    n713 = local write "Point 3 - 0.6 mm"(w779) -> ()
                    n714 = property on="Point 3 - 0.6 mm" class="Bool"("Caption.Visible"=w779) -> ()  [unwired: 2 in, 2 out]
                  }
                }
                n715 = case shown="True" w760 {
                  selector: w760 -> [w776 w777]
                  frame True {
                    n716 = local write "Point 4 - 0.8 mm"(w776) -> ()
                    n717 = property on="Point 4 - 0.8 mm" class="Bool"("Caption.Visible"=w776) -> ()  [unwired: 2 in, 2 out]
                  }
                  frame False {
                    n718 = local write "Point 4 - 0.8 mm"(w777) -> ()
                    n719 = property on="Point 4 - 0.8 mm" class="Bool"("Caption.Visible"=w777) -> ()  [unwired: 2 in, 2 out]
                  }
                }
                n720 = case shown="True" w758 {
                  selector: w758 -> [w772 w773]
                  frame True {
                    n721 = local write "Point 6 - 1.2 mm"(w772) -> ()
                    n722 = property on="Point 6 - 1.2 mm" class="Bool"("Caption.Visible"=w772) -> ()  [unwired: 2 in, 2 out]
                  }
                  frame False {
                    n723 = local write "Point 6 - 1.2 mm"(w773) -> ()
                    n724 = property on="Point 6 - 1.2 mm" class="Bool"("Caption.Visible"=w773) -> ()  [unwired: 2 in, 2 out]
                  }
                }
              }
            }
          }
        }
      }
      event "Accept & Save": Value Change {
        n725 = event-data() -> ()  [unwired: 1 in, 6 out]
        n726 = flat-sequence {
          frame #0 {
            n727 = Get Date/Time In Seconds() -> (seconds since 1Jan1904=w786:timestamp)
            n728 = Format Into String(format string="%<%m/%d/%Y %I:%M:%S %p>T", w786) -> (resulting string=w784:string)  [unwired: 2 in, 1 out]
            n729 = local write "STROKE CALIBRATION"(w784) -> ()
          }
          frame #1 {
            n730 = local write "Save Button"(TRUE ("Save Button")) -> ()
          }
          frame #2 {
            n731 = local write "MOVE CARRIAGE TO"(1.0 ("MOVE CARRIAGE TO")) -> ()
            n732 = local write "Main Calibration Tab"(T9."Main" ("Main Calibration Tab")) -> ()
            n733 = local write "Main Stroke Tab"(T11."Step 1" ("Main Stroke Tab")) -> ()
            n734 = local write "Calibration Selection"(T10."Default" ("Calibration Selection")) -> ()
            n735 = local write "Back Stroke 8"(FALSE ("Back Stroke 8")) -> ()
          }
        }
      }
      event "TEMPERATURE STEP Back 1", "TEMPERATURE STEP Back air Temp": Value Change {
        n736 = event-data() -> ()  [unwired: 1 in, 6 out]
        n737 = stacked-sequence {
          frame #0 {
            n738 = local write "Main Calibration Tab"(T9."Main" ("Main Calibration Tab")) -> ()
            n739 = local write "Tab Control 4"(T14."Main" ("Tab Control 4")) -> ()
            n740 = local write "Temperature Selection"(T15."Default" ("Temperature Selection")) -> ()
          }
          frame #1 {
            n741 = Wait (ms)(milliseconds to wait=u32 1000) -> ()  [unwired: 1 out]
            n742 = local write "Calibration Selection"(T10."Default" ("Calibration Selection")) -> ()
          }
          frame #2 {
            n743 = local write "Due Write"("CAL;END" ("Command")) -> ()
          }
          frame #3 {
            n744 = Wait (ms)(milliseconds to wait=u32 2000) -> ()  [unwired: 1 out]
          }
          frame #4 {
            n745 = local write "Due Write"("CAL;END" ("Command")) -> ()
          }
        }
      }
      event "Temperature Continue Step 1": Value Change {
        n746 = event-data() -> ()  [unwired: 1 in, 6 out]
        n747 = stacked-sequence {
          frame #0 {
            n748 = Wait (ms)(milliseconds to wait=u32 1000) -> ()  [unwired: 1 out]
          }
          frame #1 {
            n749 = local write "Due Write"("CAL;START" ("Command")) -> ()
          }
          frame #2 {
            n750 = Wait (ms)(milliseconds to wait=u32 500) -> ()  [unwired: 1 out]
          }
          frame #3 {
            n751 = local write "Due Write"("CAL;START" ("Command")) -> ()
          }
          frame #4 {
            n752 = Wait (ms)(milliseconds to wait=u32 1000) -> ()  [unwired: 1 out]
          }
          frame #5 {
          }
          frame #6 {
          }
          frame #7 {
          }
          frame #8 {
            n753 = local write "Tab Control 4"(T14."Step 2" ("Tab Control 4")) -> ()
          }
        }
      }
      event "Temperature Continue Step air Step 1": Value Change {
        n754 = event-data() -> ()  [unwired: 1 in, 6 out]
        n755 = stacked-sequence {
          frame #0 {
            n756 = Wait (ms)(milliseconds to wait=u32 1000) -> ()  [unwired: 1 out]
          }
          frame #1 {
            n757 = local write "Due Write"("CAL;START" ("Command")) -> ()
          }
          frame #2 {
            n758 = Wait (ms)(milliseconds to wait=u32 1000) -> ()  [unwired: 1 out]
          }
          frame #3 {
            n759 = local write "Due Write"("CAL;START" ("Command")) -> ()
          }
          frame #4 {
          }
          frame #5 {
          }
          frame #6 {
          }
          frame #7 {
          }
          frame #8 {
            n760 = local write "Tab Control 4"(T14."Air Step 2" ("Tab Control 4")) -> ()
          }
        }
      }
      event "Temperature Selection": Value Change {
        n761 = event-data() -> ()  [unwired: 1 in, 6 out]
        n762 = local read "Temperature Selection"() -> (w812:T15)
        n763 = case shown="\"Sample Temperature\"" w812 {
          frame "Air Temperature" {
            n764 = local write "Tab Control 4"(T14."Air Step 1" ("Tab Control 4")) -> ()
          }
          frame "Sample Temperature" {
            n765 = local write "Tab Control 4"(T14."Step 1" ("Tab Control 4")) -> ()
          }
          frame "Default", Default {
          }
        }
      }
      event "Temperature Continue Step 2": Value Change {
        n766 = event-data() -> ()  [unwired: 1 in, 6 out]
        n767 = stacked-sequence {
          frame #0 {
            n768 = stacked-sequence {
              frame #0 {
                n769 = Wait (ms)(milliseconds to wait=u32 1500) -> ()  [unwired: 1 out]
              }
              frame #1 {
                # "CAL;A1;<true_T>"
                n770 = local read "Sensor value"() -> (→"Sample 0deg temp":dbl)
                n771 = local write "Due Write"("CAL;A1;0" ("Command")) -> ()
              }
              frame #2 {
                n772 = Wait (ms)(milliseconds to wait=u32 1500) -> ()  [unwired: 1 out]
              }
              frame #3 {
                # "CAL;A1;<true_T>"
                n773 = local write "Due Write"("CAL;A1;0" ("Command")) -> ()
              }
              frame #4 {
              }
            }
          }
          frame #1 {
            n774 = local write "Tab Control 4"(T14."Step 3" ("Tab Control 4")) -> ()
          }
        }
      }
      event "Temperature Continue Air Step 2": Value Change {
        n775 = event-data() -> ()  [unwired: 1 in, 6 out]
        n776 = stacked-sequence {
          frame #0 {
            n777 = stacked-sequence {
              frame #0 {
                n778 = Wait (ms)(milliseconds to wait=u32 1000) -> ()  [unwired: 1 out]
              }
              frame #1 {
                # "CAL;A1;<true_T>"
                n779 = local write "Due Write"("CAL;A1;0" ("Command")) -> ()
              }
              frame #2 {
                n780 = Wait (ms)(milliseconds to wait=u32 1000) -> ()  [unwired: 1 out]
              }
              frame #3 {
                # "CAL;A1;<true_T>"
                n781 = local write "Due Write"("CAL;A1;0" ("Command")) -> ()
              }
              frame #4 {
                n782 = local read "Sensor value"() -> (→"Air 0deg temp":dbl)
              }
            }
